vi "RoundDBL.vi"(5 "Decimal places":i8, 6 "Number":dbl format="%#.10f") -> (2 "Rounded number":dbl format="%#.10f")   [LabVIEW 2017, in "GPNumeric.lvlib"]
doc: "Rounds <B>Number</B> to a number of <B>Decimal places</B>.\n\nYou can set <B>Decimal places</B> to a negative number to round to nearest 10, nearest 100 and so on. E.g. to round 782.402 to the nearest hundred, you set <B>Decimal places</B> to -2 and the <B>Rounded number</B> will be 800.\n\nThis VI is inlined.\n\n<B>Note</B> This VI uses the default IEEE 754 round-half-to-even rounding mode.\n\nSteen Schmidt\nGPower\n14/5 2014"
uses:
  GPNumeric.lvlib
panel:
  # "Copyright © 2014\nGPower\nSee enclosed license file for terms and conditions"
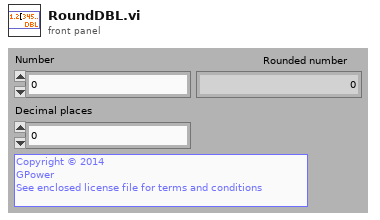
[diagram p1: front panel]
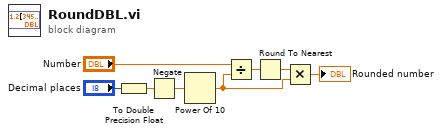
[diagram p0: block diagram]
diagram:
  n1 = To Double Precision Float(number="Decimal places") -> (double precision float=w1:dbl)
  n2 = Negate(x=w1) -> (-x=w5:dbl)
  n3 = Power Of 10(x=w5) -> (10^x=w6:dbl)
  n4 = Divide(x="Number", y=w6) -> (x/y=w8:dbl)
  n5 = Round To Nearest(number=w8) -> (nearest integer value=w7:dbl)
  n6 = Multiply(x=w7, y=w6) -> (x*y=→"Rounded number":dbl)
